vi "Module Name--constant.vi"() -> (3 "Module Name":string)   [LabVIEW 2020, in "Modulo Singleton w HL.lvlib"]
doc: "Return the name of the module that owns this VI. \n_____\nBased on Delacor QMH Project Template 5.0.0.82."
uses:
  Modulo Singleton w HL.lvlib
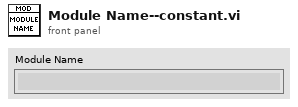
[diagram p1: front panel]
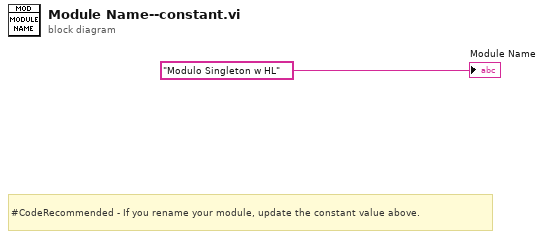
[diagram p0: block diagram]
diagram:
  # "#CodeRecommended - If you rename your module, update the constant value above."
  "Module Name" <- "Modulo Singleton w HL"
